vi "FPGA_controlled VI.vi"() -> ()   [LabVIEW 2020]
uses:
  <vilib>/rvi/Emulation/niFpgaGetClockAttributes.vi
  <vilib>/rvi/Emulation/niFpgaSctlEmulationGetInTimedLoop.vi
  <vilib>/rvi/Emulation/niFpgaEmulationReportErrorSimple.vi
  <vilib>/rvi/eio/common/nirviEmuTemplateMethod_errors.vi
  <vilib>/rvi/Emulation/niFpgaCriticalErrorInLSC.vi
  <vilib>/eio/EIONode/EIONode.xnode
panel:
  out "Mod3/DIO0":bool
  out "Mod1/AI3":fxp<+/-,26,5>
  out "Mod1/AI2":fxp<+/-,26,5>
  out "Mod1/AI1":fxp<+/-,26,5>
  in  "Mod2/AO0":fxp<+/-,20,5>
  out "Mod1/AI0":fxp<+/-,26,5>
  in  "stop":bool
  in  "Mod4/AO0":fxp<+/-,20,5>
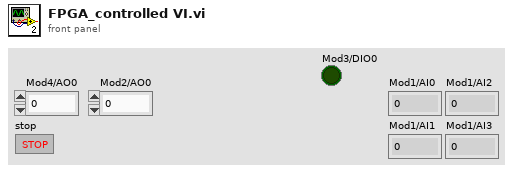
[diagram p1: front panel]
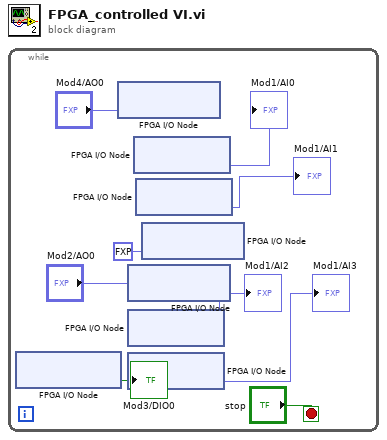
[diagram p0: block diagram]
diagram:
  n1 = while {
    stop <- "stop" stop-if-true
    n2 = xnode "FPGA I/O Node"() -> ("Mod3/DIO0"=→"Mod3/DIO0":bool)  [unwired: 1 in, 1 out]
    n3 = xnode "FPGA I/O Node"("Mod4/AO0"="Mod4/AO0") -> ()  [unwired: 1 in, 1 out]
    n4 = xnode "FPGA I/O Node"("Mod2/AO0"="Mod2/AO0") -> ()  [unwired: 1 in, 1 out]
    n5 = xnode "FPGA I/O Node"() -> ("Mod1/AI2"=→"Mod1/AI2":fxp<+/-,26,5>)  [unwired: 1 in, 1 out]
    n6 = xnode "FPGA I/O Node"() -> ("Mod1/AI3"=→"Mod1/AI3":fxp<+/-,26,5>)  [unwired: 1 in, 1 out]
    n7 = xnode "FPGA I/O Node"() -> ("Mod1/AI0"=→"Mod1/AI0":fxp<+/-,26,5>)  [unwired: 1 in, 1 out]
    n8 = xnode "FPGA I/O Node"() -> ("Mod1/AI1"=→"Mod1/AI1":fxp<+/-,26,5>)  [unwired: 1 in, 1 out]
    n9 = xnode "FPGA I/O Node"("Mod2/AO3"=fxp<+/-,20,5> 1.0) -> ()  [unwired: 1 in, 1 out]
  }
